vi "initialize_weights.vi"(2 "n[l-1]":i32, 3 "n[l]":i32) -> (0 "b":dbl[][](array[numeric]), 1 "W":dbl[][](array[numeric]))   [LabVIEW 2020]
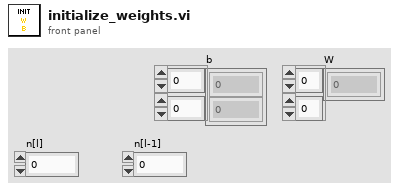
[diagram p1: front panel]
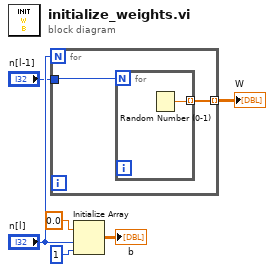
[diagram p0: block diagram]
diagram:
  n1 = for {
    N: "n[l]" -> [_]
    tunnel: "n[l-1]" -> [w8]
    tunnel: [w7] -> w2 mode=indexing
    n2 = for {
      N: w8 -> [_]
      tunnel: [w9] -> w7 mode=indexing
      n3 = Random Number (0-1)() -> (number: 0 to 1=w9:dbl)
    }
  }
  "W" <- w2
  n4 = Initialize Array(0.0 ("element"), "n[l]", 1 ("dimension size")) -> (→"b":dbl[][])
